vi "test_ort_fit.vi"() -> ()   [LabVIEW 2016]
uses:
  <vilib>/rvi/DesktopExecutionNode/Execution/niFpgaDEN_Execute.vi
  <vilib>/rvi/DesktopExecutionNode/DesktopExecutionNode.xnode
panel:
  out "expMAWave":i16[](graph)
  in  "ort.p.fcAvgEnable":bool
  out "expMATest":T1(array[cluster])
  out "dissipationGraph":dbl[](graph)
  out "dissipation":fxp<+/-,32,1>[](array[numeric])=[1.5618279576301575e-06, 1.5348196029663086e-06, 1.5399418771266937e-06, 1.505482941865921e-06, 1.4891847968101501e-06, 1.5171244740486145e-06, 1.5674158930778503e-06, 1.5636906027793884e-06, 1.5320256352424622e-06, 1.507345587015152e-06, 2.1564774215221405e-06, 2.1262094378471375e-06, 2.0260922610759735e-06, 2.1257437765598297e-06, 2.1136365830898285e-06, 2.230517566204071e-06, 1.866370439529419e-06, 2.0656734704971313e-06, 2.2151507437229156e-06, 2.032145857810974e-06]
  out "adhesions":dbl[](graph)=[-100.0, -101.0, -100.0, -102.0, -101.0, -99.0, -103.0, -103.0, -103.0, -100.0, -113.0, -117.0, -112.0, -107.0, -120.0, -113.0, -119.0, -116.0, -112.0, -104.0]
  out "debugOut":T2(array[cluster])
  out "fitBwd":T3(array[cluster])=[{"Element"={"linSum"=7691, "wtSum"=181.99217224121094, "count"=55}, 315}, {"Element"={"linSum"=7666, "wtSum"=181.2234344482422, "count"=55}, 815}, {"Element"={"linSum"=7675, "wtSum"=180.8427276611328, "count"=55}, 1315}, {"Element"={"linSum"=7679, "wtSum"=181.51412963867188, "count"=55}, 1815}, {"Element"={"linSum"=7662, "wtSum"=181.08609008789062, "count"=55}, 2315}, {"Element"={"linSum"=7674, "wtSum"=181.58975219726562, "count"=55}, 2815}, {"Element"={"linSum"=7707, "wtSum"=182.30604553222656, "count"=55}, 3315}, {"Element"={"linSum"=7703, "wtSum"=182.0128936767578, "count"=55}, 3815}, {"Element"={"linSum"=7664, "wtSum"=180.27224731445312, "count"=55}, 4315}, {"Element"={"linSum"=7677, "wtSum"=181.74880981445312, "count"=55}, 4815}, {"Element"={"linSum"=21236, "wtSum"=963.8620758056641, "count"=78}, 5338}, {"Element"={"linSum"=21220, "wtSum"=968.6760864257812, "count"=78}, 5838}, {"Element"={"linSum"=21074, "wtSum"=962.1092529296875, "count"=77}, 6337}, {"Element"={"linSum"=21237, "wtSum"=971.4603729248047, "count"=79}, 6839}, {"Element"={"linSum"=21245, "wtSum"=975.2263793945312, "count"=77}, 7337}, {"Element"={"linSum"=21227, "wtSum"=972.5785827636719, "count"=78}, 7838}, {"Element"={"linSum"=20996, "wtSum"=944.2543029785156, "count"=78}, 8338}, {"Element"={"linSum"=21100, "wtSum"=949.4695892333984, "count"=77}, 8837}, {"Element"={"linSum"=21290, "wtSum"=979.3153686523438, "count"=77}, 9337}, {"Element"={"linSum"=21022, "wtSum"=960.3946685791016, "count"=78}, 9838}]
  out "fitFwd":T3(array[cluster])=[{"Element"={"linSum"=5878, "wtSum"=93.38230895996094, "count"=46}, 306}, {"Element"={"linSum"=5908, "wtSum"=93.43618774414062, "count"=46}, 806}, {"Element"={"linSum"=5877, "wtSum"=92.73899841308594, "count"=46}, 1306}, {"Element"={"linSum"=5869, "wtSum"=93.15669250488281, "count"=46}, 1806}, {"Element"={"linSum"=5917, "wtSum"=94.27943420410156, "count"=46}, 2306}, {"Element"={"linSum"=5894, "wtSum"=93.98370361328125, "count"=46}, 2806}, {"Element"={"linSum"=5872, "wtSum"=93.11128234863281, "count"=46}, 3306}, {"Element"={"linSum"=5887, "wtSum"=93.351806640625, "count"=46}, 3806}, {"Element"={"linSum"=5886, "wtSum"=93.31344604492188, "count"=46}, 4306}, {"Element"={"linSum"=5887, "wtSum"=93.26847839355469, "count"=46}, 4806}, {"Element"={"linSum"=17607, "wtSum"=616.8370361328125, "count"=70}, 5330}, {"Element"={"linSum"=17651, "wtSum"=620.2673645019531, "count"=70}, 5830}, {"Element"={"linSum"=17568, "wtSum"=616.4625854492188, "count"=68}, 6328}, {"Element"={"linSum"=17576, "wtSum"=605.5916442871094, "count"=70}, 6830}, {"Element"={"linSum"=17460, "wtSum"=608.2845153808594, "count"=70}, 7330}, {"Element"={"linSum"=17466, "wtSum"=607.5399627685547, "count"=69}, 7829}, {"Element"={"linSum"=17699, "wtSum"=630.0108947753906, "count"=70}, 8330}, {"Element"={"linSum"=17570, "wtSum"=601.4825439453125, "count"=69}, 8829}, {"Element"={"linSum"=17566, "wtSum"=616.236083984375, "count"=69}, 9329}, {"Element"={"linSum"=17534, "wtSum"=612.8192138671875, "count"=69}, 9829}]
  in  "curveParams":T4(array[cluster])=[{"amplitude"=1000.0, "peakHeight"=200.0, "cycleLength"=500, "snapIn"=10.0, "adhesion"=100.0, "peakShift"=0, "noiseAmplitude"=2.0, "asymmetry"=0.0}, {"amplitude"=1000.0, "peakHeight"=400.0, "cycleLength"=500, "snapIn"=10.0, "adhesion"=100.0, "peakShift"=0, "noiseAmplitude"=10.0, "asymmetry"=0.2}]
  out "slopesReconvert":dbl[][](graph)=[[-2986.0, -3001.0, -2985.25, -2981.5, -3006.0, -2994.25, -2982.75, -2990.5, -2990.0, -2990.5, -2702.5, -2709.5, -2929.0, -2696.25, -2679.5, -2792.5, -2718.0, -2807.5, -2809.25, -2803.75], [-2337.5, -2329.75, -2332.25, -2333.75, -2328.5, -2332.25, -2342.25, -2341.0, -2329.0, -2333.25, -2423.25, -2422.0, -2494.25, -2338.75, -2515.25, -2423.0, -2394.75, -2495.75, -2520.75, -2399.5]]
  out "numFitEls":i32=250
  in  "fitCoeffMin":i32=1
  in  "fitCoeffMax":i32=16
  out "slopeArray":T5(array[cluster])=[{"output"={"slope"=-0.005695343017578125, "forward"=TRUE}, 314}, {"output"={"slope"=-0.004458427429199219, "forward"=FALSE}, 323}, {"output"={"slope"=-0.0057239532470703125, "forward"=TRUE}, 814}, {"output"={"slope"=-0.004443645477294922, "forward"=FALSE}, 823}, {"output"={"slope"=-0.005693912506103516, "forward"=TRUE}, 1314}, {"output"={"slope"=-0.004448413848876953, "forward"=FALSE}, 1323}, {"output"={"slope"=-0.005686759948730469, "forward"=TRUE}, 1814}, {"output"={"slope"=-0.004451274871826172, "forward"=FALSE}, 1823}, {"output"={"slope"=-0.005733489990234375, "forward"=TRUE}, 2314}, {"output"={"slope"=-0.004441261291503906, "forward"=FALSE}, 2323}, {"output"={"slope"=-0.005711078643798828, "forward"=TRUE}, 2814}, {"output"={"slope"=-0.004448413848876953, "forward"=FALSE}, 2823}, {"output"={"slope"=-0.005689144134521484, "forward"=TRUE}, 3314}, {"output"={"slope"=-0.004467487335205078, "forward"=FALSE}, 3323}, {"output"={"slope"=-0.005703926086425781, "forward"=TRUE}, 3814}, {"output"={"slope"=-0.0044651031494140625, "forward"=FALSE}, 3823}, {"output"={"slope"=-0.005702972412109375, "forward"=TRUE}, 4314}, {"output"={"slope"=-0.0044422149658203125, "forward"=FALSE}, 4323}, {"output"={"slope"=-0.005703926086425781, "forward"=TRUE}, 4814}, {"output"={"slope"=-0.004450321197509766, "forward"=FALSE}, 4823}, {"output"={"slope"=-0.005154609680175781, "forward"=TRUE}, 5338}, {"output"={"slope"=-0.004621982574462891, "forward"=FALSE}, 5346}, {"output"={"slope"=-0.005167961120605469, "forward"=TRUE}, 5838}, {"output"={"slope"=-0.004619598388671875, "forward"=FALSE}, 5846}, {"output"={"slope"=-0.0055866241455078125, "forward"=TRUE}, 6336}, {"output"={"slope"=-0.004757404327392578, "forward"=FALSE}, 6345}, {"output"={"slope"=-0.005142688751220703, "forward"=TRUE}, 6838}, {"output"={"slope"=-0.004460811614990234, "forward"=FALSE}, 6847}, {"output"={"slope"=-0.005110740661621094, "forward"=TRUE}, 7338}, {"output"={"slope"=-0.004797458648681641, "forward"=FALSE}, 7345}, {"output"={"slope"=-0.005326271057128906, "forward"=TRUE}, 7837}, {"output"={"slope"=-0.0046215057373046875, "forward"=FALSE}, 7846}, {"output"={"slope"=-0.005184173583984375, "forward"=TRUE}, 8338}, {"output"={"slope"=-0.004567623138427734, "forward"=FALSE}, 8346}, {"output"={"slope"=-0.005354881286621094, "forward"=TRUE}, 8837}, {"output"={"slope"=-0.004760265350341797, "forward"=FALSE}, 8845}, {"output"={"slope"=-0.005358219146728516, "forward"=TRUE}, 9337}, {"output"={"slope"=-0.004807949066162109, "forward"=FALSE}, 9345}, {"output"={"slope"=-0.005347728729248047, "forward"=TRUE}, 9837}, {"output"={"slope"=-0.004576683044433594, "forward"=FALSE}, 9846}]
  out "Waveform Graph":u16[](graph)
  out "paramDebug":cluster{"index":u16, "minimum":i16}[](array[cluster])
  out "minVals":T6(array[cluster])=[{{"outMinFwd"=-11.0, "outMinBwd"=-100.0}, 459}, {{"outMinFwd"=-9.0, "outMinBwd"=-101.0}, 959}, {{"outMinFwd"=-9.0, "outMinBwd"=-100.0}, 1459}, {{"outMinFwd"=-7.0, "outMinBwd"=-102.0}, 1959}, {{"outMinFwd"=-6.0, "outMinBwd"=-101.0}, 2459}, {{"outMinFwd"=-7.0, "outMinBwd"=-99.0}, 2959}, {{"outMinFwd"=-7.0, "outMinBwd"=-103.0}, 3459}, {{"outMinFwd"=-7.0, "outMinBwd"=-103.0}, 3959}, {{"outMinFwd"=-8.0, "outMinBwd"=-103.0}, 4459}, {{"outMinFwd"=-7.0, "outMinBwd"=-100.0}, 4959}, {{"outMinFwd"=-28.0, "outMinBwd"=-113.0}, 5459}, {{"outMinFwd"=-25.0, "outMinBwd"=-117.0}, 5959}, {{"outMinFwd"=-25.0, "outMinBwd"=-112.0}, 6459}, {{"outMinFwd"=-24.0, "outMinBwd"=-107.0}, 6959}, {{"outMinFwd"=-23.0, "outMinBwd"=-120.0}, 7459}, {{"outMinFwd"=-37.0, "outMinBwd"=-113.0}, 7959}, {{"outMinFwd"=-22.0, "outMinBwd"=-119.0}, 8459}, {{"outMinFwd"=-30.0, "outMinBwd"=-116.0}, 8959}, {{"outMinFwd"=-21.0, "outMinBwd"=-112.0}, 9459}, {{"outMinFwd"=-26.0, "outMinBwd"=-104.0}, 9959}] {"?"."outMinFwd" format="%.2f"; "?"."outMinBwd" format="%.2f"}
  out "Array 2":cluster{"index":u16, "data":i16}[](array[cluster])
  out "Array":bool[](array[boolean])
  out "ortCurve":dbl[](graph)
  in  "ort.p.methodParams":T7={"ort.p.winSizeP2"=2, "ort.p.syncPoint"=350, "ort.p.useSyncPoint"=TRUE, "ort.p.bypassAvg"=FALSE, "ort.p.searchBounds"={"maxSearchLower"=0, "maxSearchUpper"=0}}
  out "procVar":cluster{"cycleMax":fxp<+/-,24,16>, i32}[](array[cluster])=[{"cycleMax"=3.0, 4}, {"cycleMax"=1.0, 356}, {"cycleMax"=4.75, 856}, {"cycleMax"=2.25, 1356}, {"cycleMax"=3.75, 1856}, {"cycleMax"=4.0, 2356}, {"cycleMax"=4.5, 2856}, {"cycleMax"=2.75, 3356}, {"cycleMax"=1.5, 3856}, {"cycleMax"=4.25, 4356}, {"cycleMax"=2.75, 4856}, {"cycleMax"=-65.5, 5356}, {"cycleMax"=-68.25, 5856}, {"cycleMax"=-60.75, 6356}, {"cycleMax"=-62.75, 6856}, {"cycleMax"=-55.25, 7356}, {"cycleMax"=-64.25, 7856}, {"cycleMax"=-59.0, 8356}, {"cycleMax"=-64.0, 8856}, {"cycleMax"=-60.75, 9356}, {"cycleMax"=-62.5, 9856}]
  in  "ort.fit.p.params":T8={"maxLoc"=255, "threshold"=20, "fitHardPtLimit"=200}
  in  "repetitions":i32=10
  in  "cantileverParams":T9={"samplingRate"=62500000.0, "cantileverFreq"=500000.0, "qFactor"=2.0} {"cantileverFreq" format="%#_6p"; "samplingRate" format="%#_6p"}
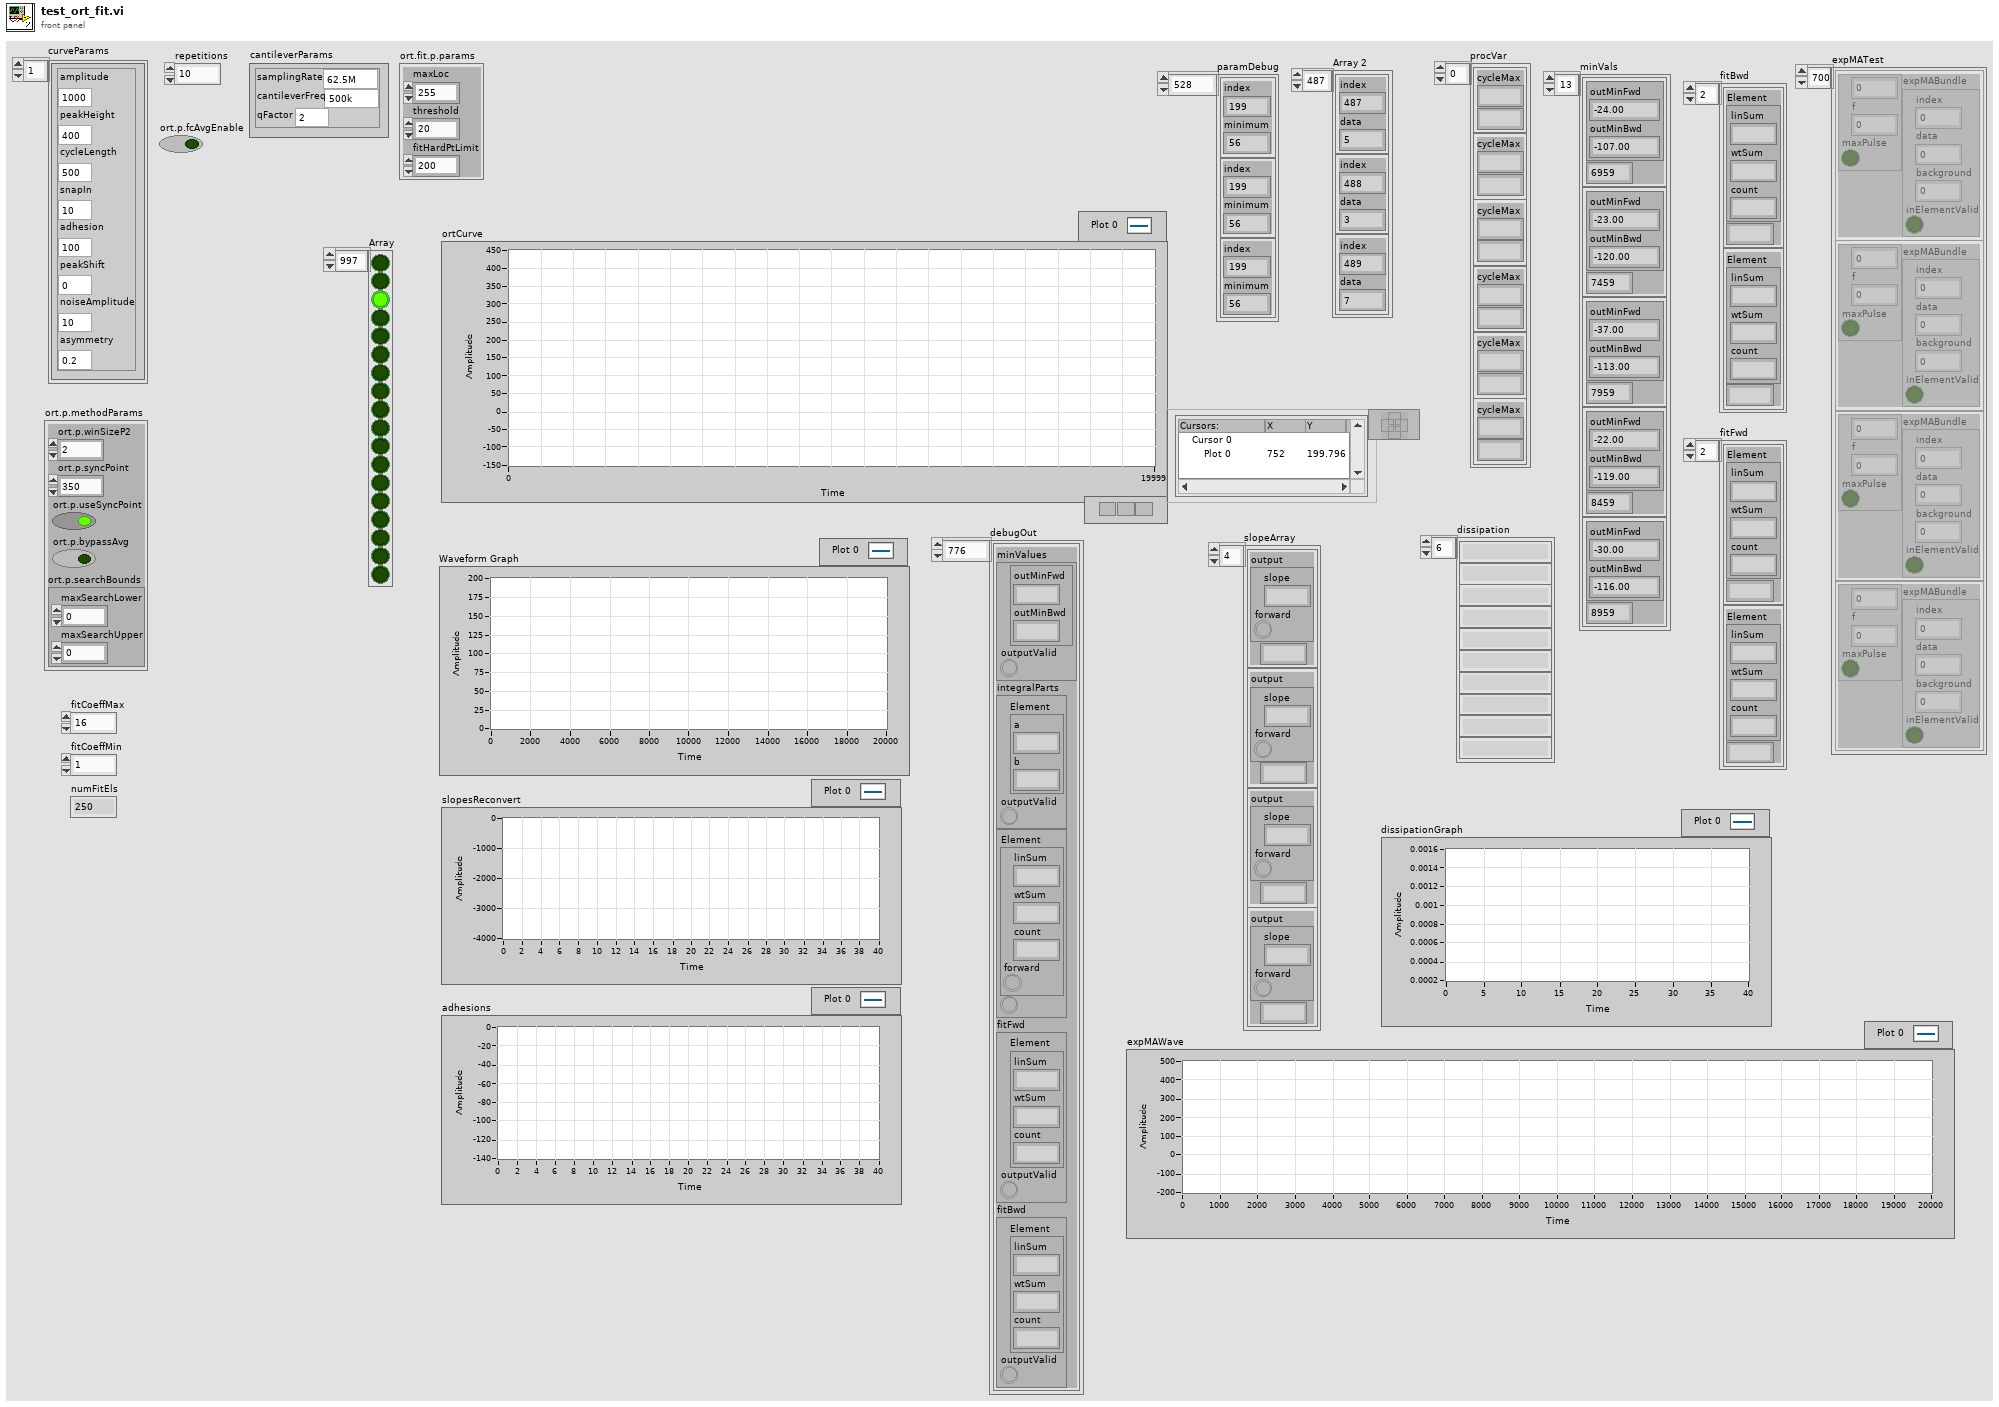
[diagram p1: front panel]
types:
  T1 = cluster{cluster{i32, "f":dbl, "maxPulse":bool}, "expMABundle":cluster{"index":u16, "data":i16, "background":i16, "inElementValid":bool}}[]
  T2 = cluster{"minValues":cluster{cluster{"outMinFwd":fxp<+/-,22,1>, "outMinBwd":fxp<+/-,22,1>}, "outputValid":bool}, "integralParts":cluster{"Element":cluster{"a":i32, "b":i32}, "outputValid":bool}, cluster{"Element":cluster{"linSum":i32, "wtSum":fxp<+/-,54,34>, "count":u16, "forward":bool}, bool}, "fitFwd":cluster{"Element":cluster{"linSum":i32, "wtSum":fxp<+/-,54,34>, "count":u16}, "outputValid":bool}, "fitBwd":cluster{"Element":cluster{"linSum":i32, "wtSum":fxp<+/-,54,34>, "count":u16}, "outputValid":bool}}[]
  T3 = cluster{"Element":cluster{"linSum":i32, "wtSum":fxp<+/-,54,34>, "count":u16}, i32}[]
  T4 = cluster{"amplitude":dbl, "peakHeight":dbl, "cycleLength":u16, "snapIn":dbl, "adhesion":dbl, "peakShift":u16, "noiseAmplitude":dbl, "asymmetry":dbl}[]
  T5 = cluster{"output":cluster{"slope":fxp<+/-,22,1>, "forward":bool}, i32}[]
  T6 = cluster{cluster{"outMinFwd":dbl, "outMinBwd":dbl}, i32}[]
  T7 = cluster{"ort.p.winSizeP2":u16, "ort.p.syncPoint":u16, "ort.p.useSyncPoint":bool, "ort.p.bypassAvg":bool, "ort.p.searchBounds":cluster{"maxSearchLower":u16, "maxSearchUpper":u16}}
  T8 = cluster{"maxLoc":u16, "threshold":i16, "fitHardPtLimit":u16}
  T9 = cluster{"samplingRate":dbl, "cantileverFreq":dbl, "qFactor":dbl}
  T10 = cluster{"write":bool, "index":u16, "fitCoefficients":cluster{"a":fxp<+/-,21,7>, "b":fxp<+/-,21,7>, "factorA":i8, "factorB":i8}}
  T11 = cluster{"write":bool, "data":fxp<+,20,0>, "index":u16}
  T12 = cluster{"amplitude":dbl, "peakHeight":dbl, "cycleLength":u16, "snapIn":dbl, "adhesion":dbl, "peakShift":u16, "noiseAmplitude":dbl, "asymmetry":dbl}
  T13 = cluster{"a":fxp<+/-,21,7>, "b":fxp<+/-,21,7>, "factorA":i8, "factorB":i8}
  T14 = cluster{"write":bool, "index":u16, "fitCoefficients":cluster{"a":fxp<+/-,21,7>, "b":fxp<+/-,21,7>, "factorA":i8, "factorB":i8}}[]
  T15 = cluster{"write":bool, "data":fxp<+,20,0>, "index":u16}[]
  T16 = cluster{cluster{"output":cluster{"slope":fxp<+/-,22,1>, "forward":bool}, "outputValid":bool}, cluster{"y":fxp<+/-,32,1>, "Output Valid":bool}}
  T17 = cluster{"cycleMax":fxp<+/-,24,16>, "maxPulse":bool}
  T18 = cluster{"minValues":cluster{cluster{"outMinFwd":fxp<+/-,22,1>, "outMinBwd":fxp<+/-,22,1>}, "outputValid":bool}, "integralParts":cluster{"Element":cluster{"a":i32, "b":i32}, "outputValid":bool}, cluster{"Element":cluster{"linSum":i32, "wtSum":fxp<+/-,54,34>, "count":u16, "forward":bool}, bool}, "fitFwd":cluster{"Element":cluster{"linSum":i32, "wtSum":fxp<+/-,54,34>, "count":u16}, "outputValid":bool}, "fitBwd":cluster{"Element":cluster{"linSum":i32, "wtSum":fxp<+/-,54,34>, "count":u16}, "outputValid":bool}}
  T19 = cluster{"index":u16, "data":i16, "background":i16, "inElementValid":bool}
  T20 = cluster{"output":cluster{"slope":fxp<+/-,22,1>, "forward":bool}, "outputValid":bool}
  T21 = cluster{cluster{"outMinFwd":fxp<+/-,22,1>, "outMinBwd":fxp<+/-,22,1>}, "outputValid":bool}
  T22 = cluster{"Element":cluster{"linSum":i32, "wtSum":fxp<+/-,54,34>, "count":u16}, "outputValid":bool}
  T23 = cluster{"outMinFwd":fxp<+/-,22,1>, "outMinBwd":fxp<+/-,22,1>}
  T24 = cluster{"linSum":i32, "wtSum":fxp<+/-,54,34>, "count":u16}
  T25 = cluster{"Element":cluster{"linSum":i32, "wtSum":fxp<+/-,54,34>, "count":u16}, i32}
  T26 = cluster{"output":cluster{"slope":fxp<+/-,22,1>, "forward":bool}, i32}
  T27 = cluster{cluster{"outMinFwd":dbl, "outMinBwd":dbl}, i32}
  T28 = cluster{cluster{i32, "f":dbl, bool}, "expMABundle":cluster{"index":u16, "data":i16, "background":i16, "inElementValid":bool}}
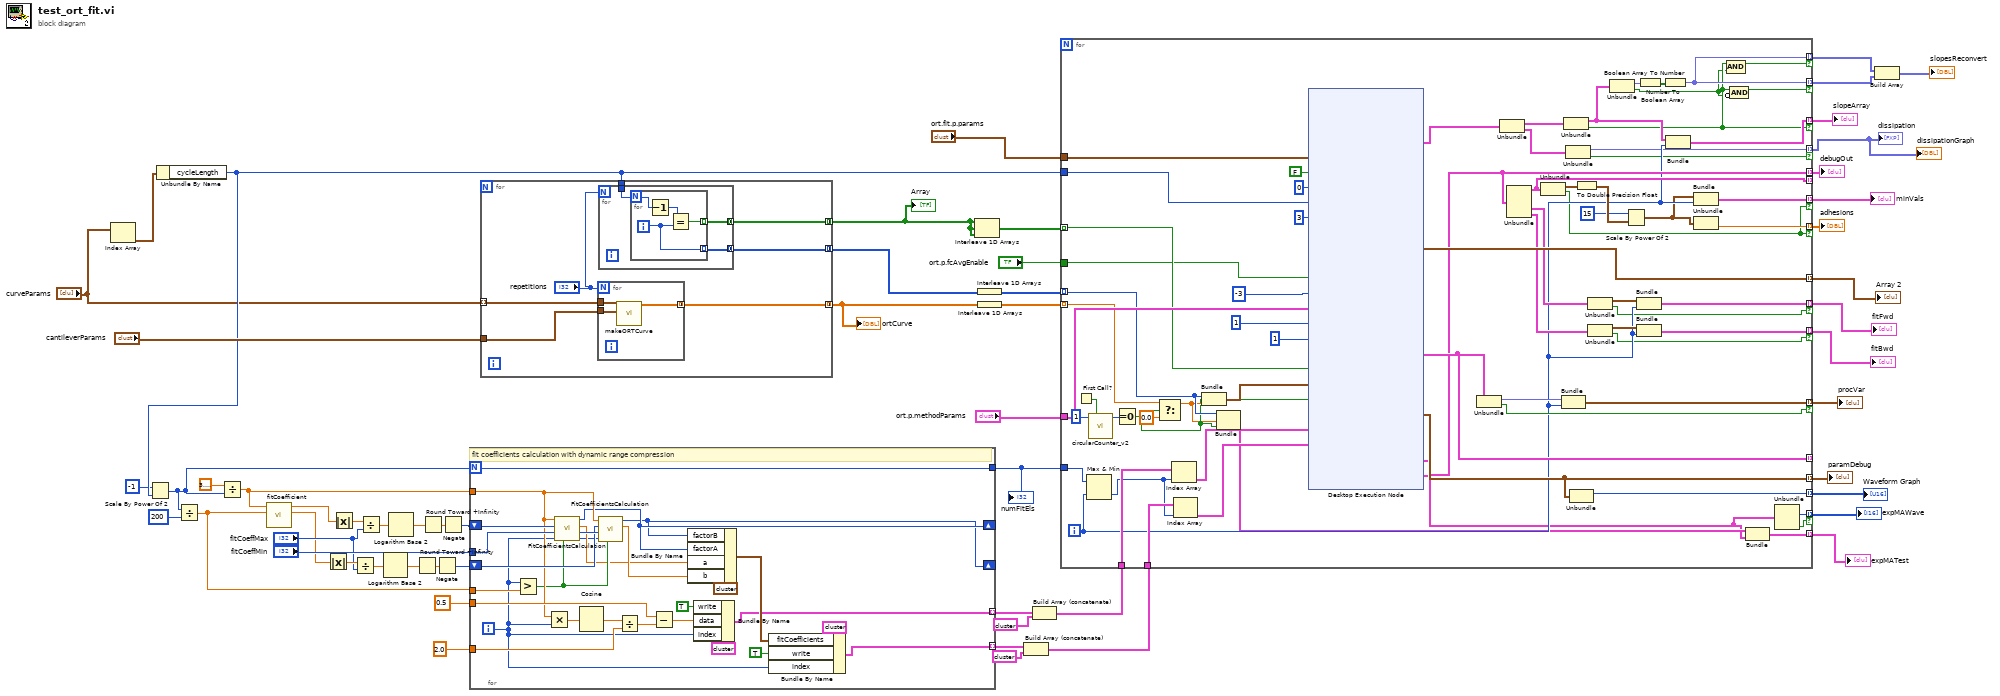
[diagram p0: block diagram]
diagram:
  n1 = Index Array(array="curveParams") -> (element=w18:T12)  [unwired: 1 in]
  n2 = Unbundle By Name(w18) -> ("cycleLength"=w49:u16)
  n3 = Scale By Power Of 2(n=i16 -1, x=w49) -> (x*2^n=w38:u16)
  n4 = Divide(x=w38, y=200) -> (x/y=w36:dbl)
  n5 = Divide(x=3.141592653589793, y=w38) -> (x/y=w47:dbl)
  n6 = call "fitCoefficient.vi"("n"=w36, "a"=w47) -> ("d"=w28:dbl, "c"=w46:dbl)  [unwired: 8 in]
  n7 = Absolute Value(x=w28) -> (abs(x)=w33:dbl)
  n8 = Absolute Value(x=w46) -> (abs(x)=w41:dbl)
  n9 = Divide(x=w33, y="fitCoeffMax") -> (x/y=w30:dbl)
  n10 = Divide(x=w41, y="fitCoeffMax") -> (x/y=w45:dbl)
  n11 = Logarithm Base 2(1:w30) -> (0:w31:dbl)
  n12 = Logarithm Base 2(1:w45) -> (0:w44:dbl)
  n13 = Round Toward +Infinity(x=w31) -> (ceil(x): smallest int >= x=w32:dbl)
  n14 = Round Toward +Infinity(x=w44) -> (ceil(x): smallest int >= x=w43:dbl)
  n15 = Negate(x=w32) -> (-x=w27:i16)
  n16 = Negate(x=w43) -> (-x=w40:i16)
  n17 = for {
    N: w38 -> [w59]
    tunnel: w47 -> [w75]
    shift-right: [w64] -> _
    shift-left: w40 -> [w84]
    tunnel: "fitCoeffMin" -> [w77]
    tunnel: w36 -> [w83]
    tunnel: 2.0 ("y") -> [w79]
    tunnel: 0.5 ("x") -> [w78]
    shift-right: [w63] -> _
    shift-left: w27 -> [w76]
    tunnel: [w61] -> w26 mode=indexing
    tunnel: [w60] -> w24 mode=indexing
    tunnel: [w59] -> w20
    i -> [w65]
    # "fit coefficients calculation with dynamic range compression"
    n18 = Greater?(x=w65, y=w83) -> (0:w74:bool)
    n19 = Multiply(x=w75, y=w65) -> (x*y=w82:dbl)
    n20 = call "FitCoefficientsCalculation.vi"("Iteration > 1/200*arraySize"=w74, "Iteration"=w65, "fitCoeffMin"=w77, "Numeric 4"=w84, "Pi/ArraySize"=w75) -> ("fitCoefficients.a-b"=w66:dbl, "fitCoefficients.Factor"=w64:i16)  [unwired: 5 in]
    n21 = Cosine(x=w82) -> (cos(x)=w81:dbl)
    n22 = call "FitCoefficientsCalculation.vi"("Iteration > 1/200*arraySize"=w74, "Iteration"=w65, "fitCoeffMin"=w77, "Numeric 4"=w76, "Pi/ArraySize"=w75) -> ("fitCoefficients.a-b"=w67:dbl, "fitCoefficients.Factor"=w63:i16)  [unwired: 5 in]
    n23 = Divide(x=w81, y=w79) -> (x/y=w80:dbl)
    n24 = Subtract(x=w78, y=w80) -> (x-y=w71:dbl)
    n25 = Bundle By Name(cluster=T13 {"a"=0.0, "b"=0.0, "factorA"=0, "factorB"=0} ("fitCoefficients"), "factorB"=w63, "factorA"=w64, "a"=w66, "b"=w67) -> (w62:T13)
    n26 = Bundle By Name(cluster=T11 {"write"=FALSE, "data"=0.0, "index"=0} ("ort.fit.m.weights"), "write"=TRUE, "data"=w71, "index"=w65) -> (w61:T11)
    n27 = Bundle By Name(cluster=T10 {"write"=FALSE, "index"=0, "fitCoefficients"={"a"=0.0, "b"=0.0, "factorA"=0, "factorB"=0}} ("ort.fit.m.coefficients"), "fitCoefficients"=w62, "write"=TRUE, "index"=w65) -> (w60:T10)
  }
  "numFitEls" <- w20
  n28 = for {
    tunnel: "cantileverParams" -> [w91]
    tunnel: [w90] -> w8 mode=concatenating
    tunnel: "curveParams" -> [w89] mode=indexing
    tunnel: [w87] -> w4 mode=concatenating
    tunnel: [w86] -> w6 mode=concatenating
    tunnel: w49 -> [w85]
    n29 = for {
      N: "repetitions" -> [_]
      tunnel: w89 -> [w101]
      tunnel: w91 -> [w100]
      tunnel: [w99] -> w90 mode=concatenating
      n30 = call "makeORTCurve.vi"("cantileverParams"=w100, "curveParams"=w101) -> ("ortCurve"=w99:dbl[])  [unwired: 9 in]
    }
    n31 = for {
      N: "repetitions" -> [_]
      tunnel: w85 -> [w94]
      tunnel: [w93] -> w87 mode=concatenating
      tunnel: [w92] -> w86 mode=concatenating
      n32 = for {
        N: w94 -> [w98]
        tunnel: [w96] -> w93 mode=indexing
        tunnel: [w95] -> w92 mode=indexing
        i -> [w95]
        n33 = Decrement(x=w98) -> (x-1=w97:i32)
        n34 = Equal?(x=w97, y=w95) -> (x = y?=w96:bool)
      }
    }
  }
  "ortCurve" <- w8
  "Array" <- w4
  n35 = Interleave 1D Arrays(w4, w4, w4) -> (w5:bool[])
  n36 = Interleave 1D Arrays(w6) -> (w7:i32[])
  n37 = Interleave 1D Arrays(w8) -> (w9:dbl[])
  n38 = Build Array (concatenate)(w24, T10 {"write"=FALSE, "index"=0, "fitCoefficients"={"a"=0.0, "b"=0.0, "factorA"=0, "factorB"=0}} ("ort.fit.m.coefficients")) -> (w21:T14)
  n39 = Build Array (concatenate)(w26, T11 {"write"=FALSE, "data"=0.0, "index"=0} ("ort.fit.m.weights")) -> (w22:T15)
  n40 = for {
    tunnel: w9 -> [w155] mode=indexing
    tunnel: "ort.fit.p.params" -> [w169]
    tunnel: [w167] -> w56 mode=indexing if=w166
    tunnel: w49 -> [w165]
    tunnel: "ort.p.methodParams" -> [w159]
    tunnel: w5 -> [w158] mode=indexing
    tunnel: w7 -> [w112] mode=indexing
    tunnel: [w157] -> _ mode=indexing
    tunnel: [w156] -> w54 mode=indexing
    tunnel: [w135] -> w15 mode=indexing
    tunnel: [w154] -> w53 mode=indexing if=w123
    tunnel: [w153] -> w52 mode=indexing
    tunnel: [w152] -> w51 mode=indexing
    tunnel: [w151] -> _ mode=indexing
    tunnel: [w145] -> w50 mode=indexing if=w118
    tunnel: w22 -> [w144]
    tunnel: w21 -> [w142]
    tunnel: w20 -> [w140]
    tunnel: [w119] -> w12 mode=indexing if=w116
    tunnel: [w129] -> w17 mode=indexing if=w127
    tunnel: [w128] -> w16 mode=indexing if=w126
    tunnel: [w124] -> w14 mode=indexing if=w123
    tunnel: [w121] -> w10 mode=indexing if=w120
    tunnel: [w119] -> w13 mode=indexing if=w117
    tunnel: [w109] -> w3 mode=indexing
    tunnel: "ort.p.fcAvgEnable" -> [w108]
    tunnel: [w103] -> w1 mode=indexing if=w102
    i -> [w130]
    n41 = First Call?() -> (First Call?: T/F=w105:bool)
    n42 = Max & Min(x=w140, y=w130) -> (min(x,y)=w139:i32)  [unwired: 1 out]
    n43 = call "circularCounter_v2.vi"("reset"=w105, "maxCount"=u16 1) -> ("index"=w107:u16)  [unwired: 6 in, 3 out]
    n44 = Equal To 0?(x=w107) -> (x = 0?=w106:bool)
    n45 = Select(t=w155, s=w106, f=0.0) -> (s? t:f=w111:dbl)
    n46 = Index Array(array=w144, index=w139) -> (element=w143:T11)
    n47 = Index Array(array=w142, index=w139) -> (element=w141:T10)
    n48 = Bundle(w112, "f"=w111) -> (w171:cluster{i32, "f":dbl})  [unwired: 1 in]
    n49 = Bundle(w112, "f"=w111, w106) -> (w110:cluster{i32, "f":dbl, bool})  [unwired: 1 in]
    n50 = xnode "Desktop Execution Node"("ort.fit.p.params"=w169, "auxInValid"=FALSE, "auxIn"=i16 0, "ort.p.waveSize"=w165, "ort.bgc.p.bgCntP2"=u16 3, "ort.p.fcAvgEnable"=w108, "ort.p.fcAvg"=i8 -3, "ort.p.methodParams"=w159, "fb.i.source"=u8 1, "aio.i.samplingDecimation"=u16 1, "endOfCycle"=w158, "inElement"=w171, "inElementValid"=w106, "ort.fit.m.weights"=w143, "ort.fit.m.coefficients"=w141) -> ("debugOutSlopeDissi"=w147:T16, "aio.s.ortSubstDeflection"=w156:cluster{"index":u16, "data":i16}, "procVar"=w157:T17, "paramExtractDebug"=w153:cluster{"index":u16, "minimum":i16}, "debugOutFitIntermediate"=w135:T18, "expMABundle"=w104:T19)  [unwired: 1 in, 3 out]
    n51 = Unbundle(w157) -> ("cycleMax"=w168:fxp<+/-,24,16>, "maxPulse"=w166:bool)
    n52 = Unbundle(w147) -> (w146:T20, w122:cluster{"y":fxp<+/-,32,1>, "Output Valid":bool})
    n53 = Unbundle(w135) -> ("minValues"=w151:T21, "fitFwd"=w134:T22, "fitBwd"=w133:T22)  [unwired: 2 out]
    n54 = Unbundle(w151) -> (w150:T23, "outputValid"=w123:bool)
    n55 = Bundle("cycleMax"=w168, w130) -> (w167:cluster{"cycleMax":fxp<+/-,24,16>, i32})  [unwired: 1 in]
    n56 = Unbundle(w146) -> ("output"=w138:cluster{"slope":fxp<+/-,22,1>, "forward":bool}, "outputValid"=w118:bool)
    n57 = Unbundle(w122) -> ("y"=w121:fxp<+/-,32,1>, "Output Valid"=w120:bool)
    n58 = Unbundle(w153) -> ("index"=w152:u16)  [unwired: 1 out]
    n59 = To Double Precision Float(number=w150) -> (double precision float=w149:cluster{"outMinFwd":dbl, "outMinBwd":dbl})
    n60 = Unbundle(w134) -> ("Element"=w132:T24, "outputValid"=w127:bool)
    n61 = Unbundle(w133) -> ("Element"=w131:T24, "outputValid"=w126:bool)
    n62 = Unbundle(w138) -> ("slope"=w137:fxp<+/-,22,1>, "forward"=w115:bool)
    n63 = Scale By Power Of 2(n=i16 15, x=w149) -> (x*2^n=w125:cluster{"outMinFwd":dbl, "outMinBwd":dbl})
    n64 = Bundle("Element"=w132, w130) -> (w129:T25)  [unwired: 1 in]
    n65 = Bundle("Element"=w131, w130) -> (w128:T25)  [unwired: 1 in]
    n66 = Number To Boolean Array(number=w137) -> (Boolean array=w136:bool[])
    n67 = Boolean Array To Number(Boolean array=w136) -> (number=w119:fxp<+/-,22,20>)
    n68 = Bundle("output"=w138, w130) -> (w145:T26)  [unwired: 1 in]
    n69 = Bundle(w125, w130) -> (w154:T27)  [unwired: 1 in]
    n70 = Unbundle(w125) -> ("outMinBwd"=w124:dbl)  [unwired: 1 out]
    n71 = Compound Arithmetic op=AND(w118, w115) -> (w117:bool)
    n72 = Compound Arithmetic op=AND(w118, invert w115) -> (w116:bool)
    n73 = Bundle(w110, "expMABundle"=w104) -> (w109:T28)  [unwired: 1 in]
    n74 = Unbundle(w104) -> ("data"=w103:i16, "inElementValid"=w102:bool)  [unwired: 2 out]
  }
  "procVar" <- w56
  "Array 2" <- w54
  "minVals" <- w53
  "paramDebug" <- w52
  "Waveform Graph" <- w51
  "slopeArray" <- w50
  "fitFwd" <- w17
  "fitBwd" <- w16
  "debugOut" <- w15
  "adhesions" <- w14
  "dissipation" <- w10
  "dissipationGraph" <- w10
  "expMATest" <- w3
  "expMAWave" <- w1
  n75 = Build Array(w13, w12) -> (→"slopesReconvert":fxp<+/-,22,20>[][])
